vi "GoToAngle.vi"(9 "Target Angle":dbl, 10 "Angle":dbl, 11 "Inverted":bool) -> (0 "AtTarget":bool, 3 "X axis":dbl)   [LabVIEW 2017]
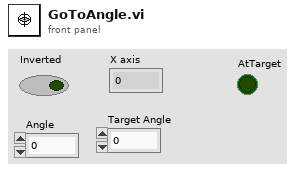
[diagram p1: front panel]
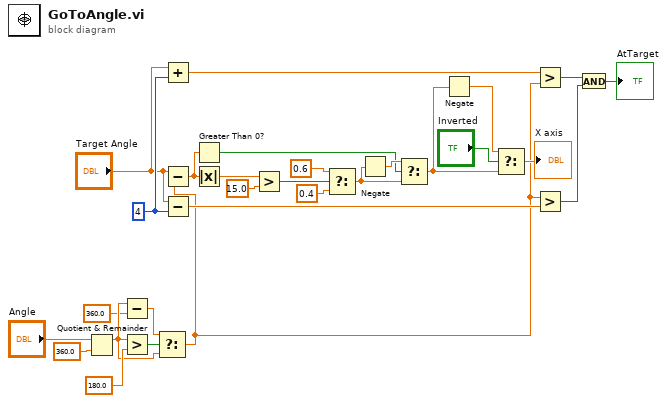
[diagram p0: block diagram]
diagram:
  w26 = 4
  n1 = Quotient & Remainder(x="Angle", y=360.0) -> (x-y*floor(x/y)=w3:dbl)  [unwired: 1 out]
  n2 = Subtract(x=w3, y=360.0) -> (x-y=w4:dbl)
  n3 = Greater?(x=w3, y=180.0) -> (0:w6:bool)
  n4 = Select(t=w4, s=w6, f=w3) -> (s? t:f=w1:dbl)
  n5 = Add(x="Target Angle", y=w26) -> (x+y=w23:dbl)
  n6 = Subtract(x="Target Angle", y=w1) -> (x-y=w11:dbl)
  n7 = Subtract(x="Target Angle", y=w26) -> (x-y=w24:dbl)
  n8 = Greater Than 0?(x=w11) -> (x > 0?=w12:bool)
  n9 = Absolute Value(x=w11) -> (abs(x)=w19:dbl)
  n10 = Greater?(x=w19, y=15.0) -> (0:w17:bool)
  n11 = Select(t=0.6, s=w17, f=0.4) -> (s? t:f=w13:dbl)
  n12 = Negate(x=w13) -> (-x=w14:dbl)
  n13 = Select(t=w14, s=w12, f=w13) -> (s? t:f=w10:dbl)
  n14 = Negate(x=w10) -> (-x=w28:dbl)
  n15 = Select(t=w28, s="Inverted", f=w10) -> (s? t:f=→"X axis":dbl)
  n16 = Greater?(x=w23, y=w1) -> (0:w21:bool)
  n17 = Greater?(x=w1, y=w24) -> (0:w22:bool)
  n18 = And(x=w21, y=w22) -> (x .and. y?=→"AtTarget":bool)
